vi "nican_loop.vi"(0 "ObjHandle A":T1, 1 "Error in A":errorcluster, 2 "ObjHandle B":T1, 3 "Error in B":errorcluster) -> (5 "Error out A":errorcluster, 6 "2D Array":u8[][](array[numeric]), 7 "Error out B":errorcluster)   [LabVIEW 2017]
uses:
  <vilib>/nican/nican.llb/xobjhandle.ctl
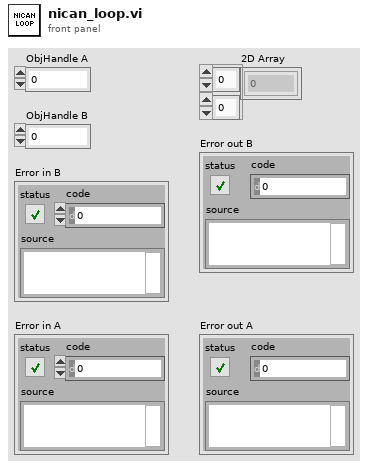
[diagram p1: front panel]
types:
  T1 = typedef "xobjhandle.ctl" = u32
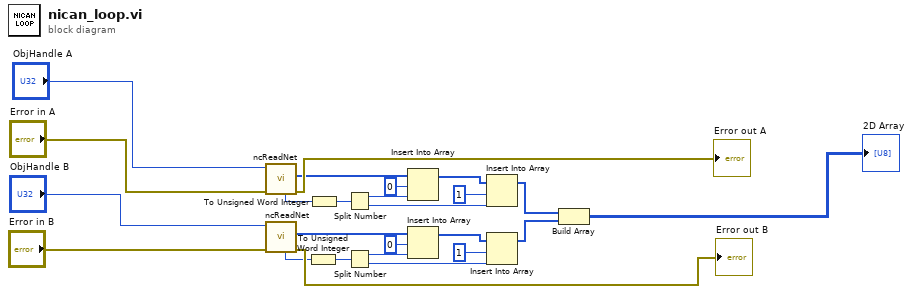
[diagram p0: block diagram]
diagram:
  n1 = call <vilib>:"ncReadNet.vi"("ObjHandle in"="ObjHandle A", "Error in"="Error in A") -> ("ArbitrationId"=w10:u32, "Data"=w14:u8[], "Error out"=→"Error out A":errorcluster)  [unwired: 2 in, 4 out]
  n2 = call <vilib>:"ncReadNet.vi"("ObjHandle in"="ObjHandle B", "Error in"="Error in B") -> ("ArbitrationId"=w4:u32, "Data"=w8:u8[], "Error out"=→"Error out B":errorcluster)  [unwired: 2 in, 4 out]
  n3 = To Unsigned Word Integer(number=w4) -> (unsigned 16bit integer=w3:u16)
  n4 = To Unsigned Word Integer(number=w10) -> (unsigned 16bit integer=w9:u16)
  n5 = Split Number(x=w9) -> (hi(x)=w12:u8, lo(x)=w11:u8)
  n6 = Split Number(x=w3) -> (hi(x)=w6:u8, lo(x)=w5:u8)
  n7 = Insert Into Array(array=w14, index=0, new element=w12) -> (w13:u8[])
  n8 = Insert Into Array(array=w8, index=0, new element=w6) -> (w7:u8[])
  n9 = Insert Into Array(array=w13, index=1, new element=w11) -> (w2:u8[])
  n10 = Insert Into Array(array=w7, index=1, new element=w5) -> (w1:u8[])
  n11 = Build Array(w2, w1) -> (→"2D Array":u8[][])
